vi "DSF.Execution.Builder.Get Plugin Buffer Pools.vi"(8 "error in (no error)":errorcluster, 11 "Builder in":refnum<class "DSF.Execution.Builder.lvclass">) -> (0 "error out":errorcluster, 2 "Plugin Buffer Pools":refnum<class "DSF.Memory.BufferPool.lvclass">[](array[class]), 3 "Builder out":refnum<class "DSF.Execution.Builder.lvclass">)   [LabVIEW 2016, in "DSF.Execution.lvlib" / "DSF.Execution.Builder.lvclass"]
uses:
  DSF.Execution.Builder.lvclass
  Memory.BufferPool/DSF.Memory.BufferPool.lvclass
  DSF.Execution.Builder.lvclass/DSF.Execution.Builder.ctl
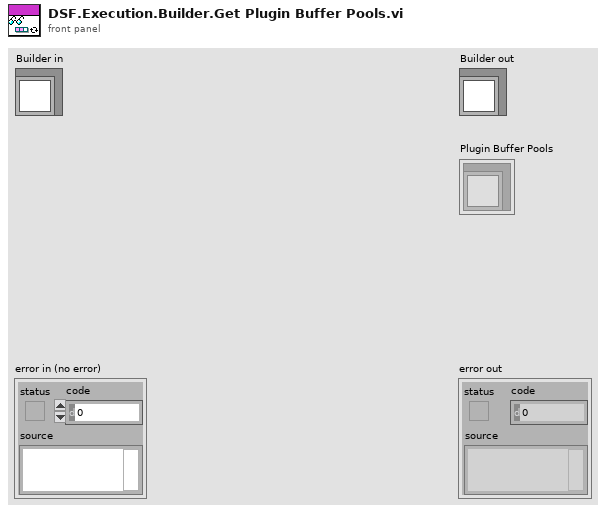
[diagram p1: front panel]
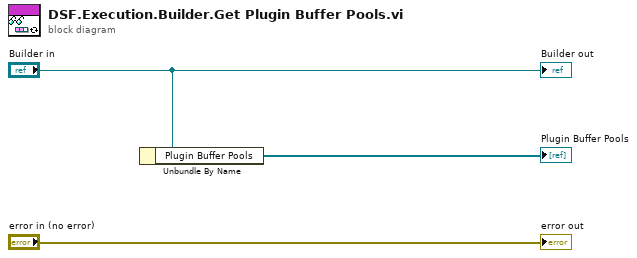
[diagram p0: block diagram]
diagram:
  n1 = Unbundle By Name("Builder in") -> ("Plugin Buffer Pools"=→"Plugin Buffer Pools":refnum<class "DSF.Memory.BufferPool.lvclass">[])
  "error out" <- "error in (no error)"
  "Builder out" <- "Builder in"
